vi "64IN_4 WaitInId.vi"(6 "time(0.1)":i32=100, 8 "error in":errorcluster, 9 "Wait?":bool=TRUE, 10 "Status":bool, 11 "64IIN_4 Select":T1) -> (0 "error Out":errorcluster, 2 "TimeOut":bool, 3 "StatusOut":bool)   [LabVIEW 2019]
uses:
  Ctrl/DMC1000B_1 SelectIn.ctl
  global/InAndOutGB.vi
  global/IO_FlagGB.vi
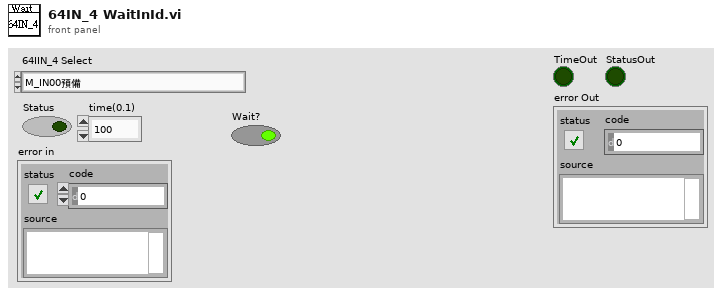
[diagram p1: front panel]
types:
  T1 = typedef "DMC1000B_1 SelectIn.ctl" = enum16{"M_IN00預備", "M_IN01緊急急停檢測", "M_IN02啟動按鈕綠色", "M_IN03正壓氣壓檢知", "M_IN04安全門感知", "M_IN05接受前機台有料#1信號", "M_IN06接受前機台有料#2信號", "M_IN07接受後機台要料#3信號", "M_IN08接受後機台要料#4信號", "M_IN09軌道載板前進料到位檢知", "M_IN10到料阻擋氣缸上位檢知(阻擋位)", "M_IN11到料阻擋氣缸下位檢知(阻擋位)", "M_IN12上頂固定載板氣缸上位檢知", "M_IN13上頂固定載板氣缸下位檢知", "M_IN14軌道載板到位減速檢知", "M_IN15軌道載板到位檢知", "M_IN16軌道載板後出料檢知", "M_IN17", "M_IN18", "M_IN19", "M_IN20", "M_IN21第一軸準備輸入信號 RDY", "M_IN22第二軸準備輸入信號 RDY", "M_IN23第三軸準備輸入信號 RDY", "M_IN24", "M_IN25第一軸ALM+(  伺服警報輸出  )", "M_IN26第二軸ALM+(  伺服警報輸出  )", "M_IN27第三軸ALM+(  伺服警報輸出  )", "M_IN28", "M_IN29第一軸定位完成信號 INP", "M_IN30第二軸定位完成信號 INP", "M_IN31第三軸定位完成信號 INP", "M_IN32"}
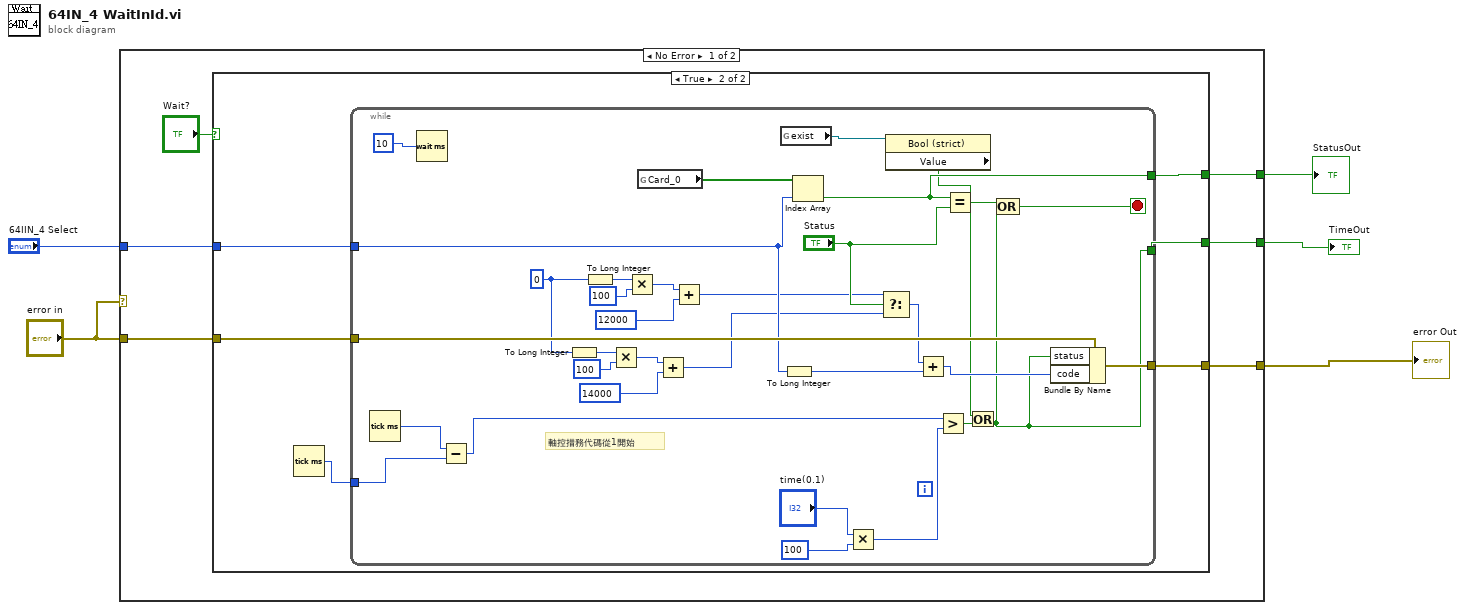
[diagram p0: block diagram]
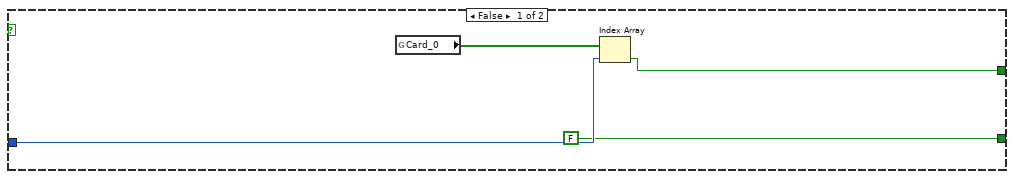
[diagram p2: hidden frame]
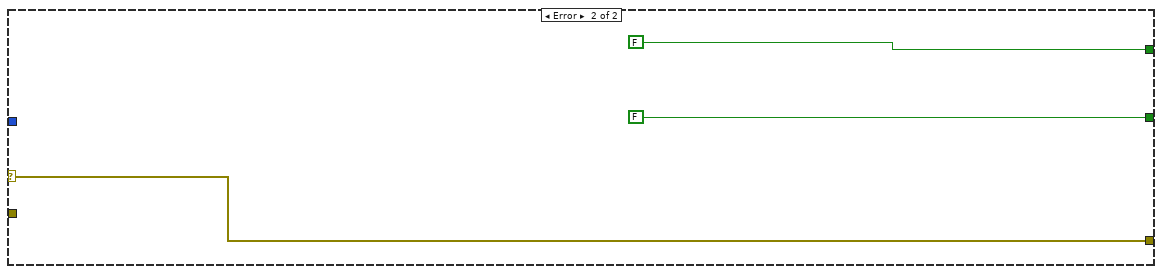
[diagram p3: hidden frame]
diagram:
  n1 = case shown="No Error" "error in" {
    selector: "error in" -> [_ w56]
    tunnel: [w11 FALSE] -> w5
    tunnel: "error in" -> [w10 _]
    tunnel: [w9 w56] -> w4
    tunnel: [w8 FALSE ("Boolean")] -> w2
    tunnel: "64IIN_4 Select" -> [w6 _]
    frame No Error {
      n2 = case shown="True" "Wait?" {
        tunnel: [FALSE w21] -> w11
        tunnel: w10 -> [_ w20]
        tunnel: [_ w19] -> w9
        tunnel: [w14 w18] -> w8
        tunnel: w6 -> [w15 w17]
        frame False {
          n3 = global read "InAndOutGB.vi" "Card_0"() -> (w12:bool[])
          n4 = Index Array(array=w12, index=w15) -> (element=w14:bool)
        }
        frame True {
          n5 = Tick Count (ms)() -> (millisecond timer value=w16:u32)
          n6 = while {
            tunnel: [w43] -> w21
            tunnel: w20 -> [w50]
            tunnel: [w47] -> w19
            tunnel: [w42] -> w18
            tunnel: w17 -> [w40]
            tunnel: w16 -> [w24]
            stop <- w52 stop-if-true
            w22 = 0 ("number")
            # "軸控措務代碼從1開始"
            n7 = Tick Count (ms)() -> (millisecond timer value=w25:u32)
            n8 = Wait (ms)(milliseconds to wait=u32 10) -> ()  [unwired: 1 out]
            n9 = Subtract(x=w25, y=w24) -> (x-y=w23:u32)
            n10 = To Long Integer(number=w22) -> (32bit integer=w30:i32)
            n11 = To Long Integer(number=w22) -> (32bit integer=w38:i32)
            n12 = Multiply(x=w30, y=100) -> (x*y=w32:i32)
            n13 = Multiply(x=w38, y=100) -> (x*y=w36:i32)
            n14 = global read "InAndOutGB.vi" "Card_0"() -> (w53:bool[])
            n15 = Add(x=w32, y=14000) -> (x+y=w29:i32)
            n16 = Add(x=w36, y=12000) -> (x+y=w34:i32)
            n17 = global read "IO_FlagGB.vi" "exist"() -> (w39:refnum<vi>)
            n18 = To Long Integer(number=w40) -> (32bit integer=w44:i32)
            n19 = Index Array(array=w53, index=w40) -> (element=w42:bool)
            n20 = Multiply(x="time(0.1)", y=u32 100 ("milliseconds to wait")) -> (x*y=w26:u32)
            n21 = Select(t=w34, s="Status", f=w29) -> (s? t:f=w45:i32)
            n22 = property class="Bool (strict)"(reference=w39) -> ("Value"=w41:bool)  [unwired: 1 in, 2 out]
            n23 = Add(x=w45, y=w44) -> (x+y=w48:i32)
            n24 = Greater?(x=w23, y=w26) -> (0:w49:bool)
            n25 = Equal?(x=w42, y="Status") -> (x = y?=w51:bool)
            n26 = Or(x=w41, y=w49) -> (x .or. y?=w43:bool)
            n27 = Compound Arithmetic op=OR(w51, w43) -> (w52:bool)
            n28 = Bundle By Name(cluster=w50, "status"=w43, "code"=w48) -> (w47:errorcluster)
          }
        }
      }
    }
    frame Error {
    }
  }
  "TimeOut" <- w5
  "error Out" <- w4
  "StatusOut" <- w2
